vi "_FP Cntrl Manager.vi"(0 "Cluster":T1, 5 "Error IN":errorcluster, 8 "Action":T2) -> (19 "Error OUT":errorcluster)   [LabVIEW 2011]
uses:
  Controls/FP Ref Enum.ctl
  Controls/FP Ref Cluster.ctl
  Program Control/RS485 Settings Top Level.ctl
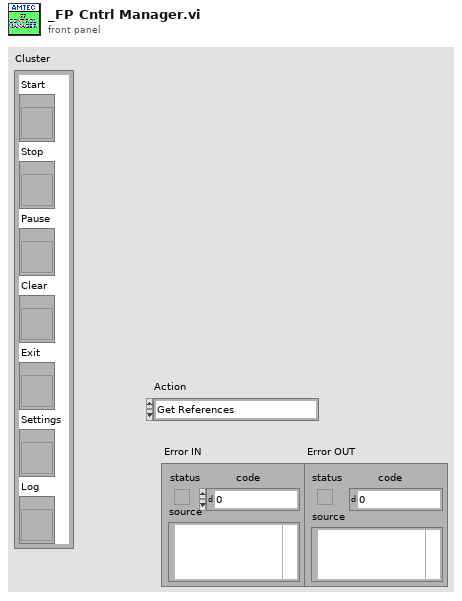
[diagram p1: front panel]
types:
  T1 = typedef "FP Ref Cluster.ctl" = cluster{"Start":refnum<vi>, "Stop":refnum<vi>, "Pause ":refnum<vi>, "Clear":refnum<vi>, "Exit":refnum<vi>, "Settings":refnum<vi>, "Log":refnum<vi>}
  T2 = typedef "FP Ref Enum.ctl" = enum16{"Get References", "Status", "Init", "Start Recording", "Stop Recording", "Pause Update", "Resume Update"}
  T3 = enum8{"Enabled", "Disabled", "Disabled and Grayed Out"}
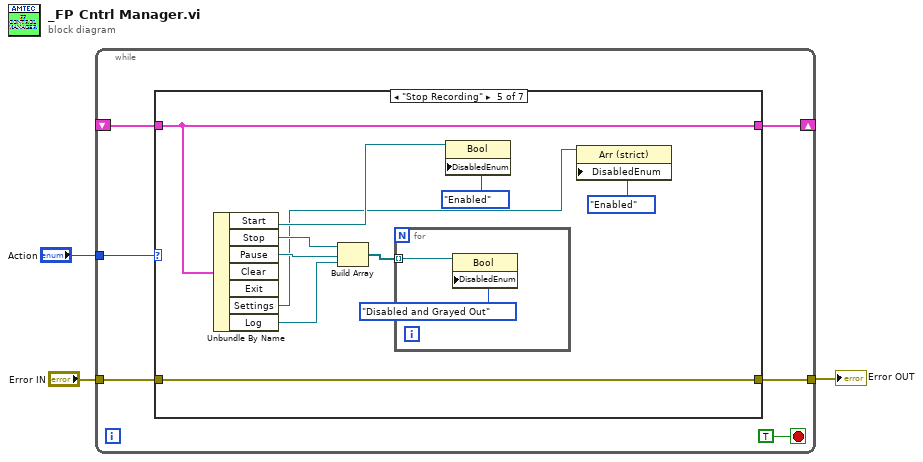
[diagram p0: block diagram]
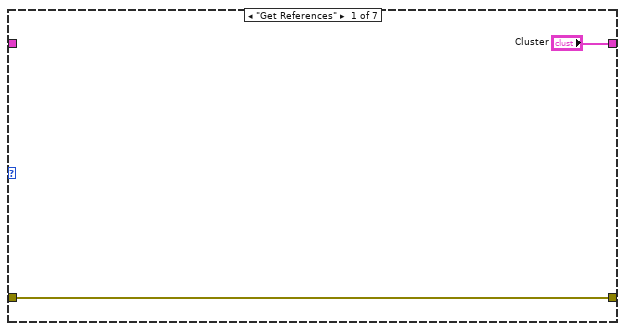
[diagram p2: hidden frame]
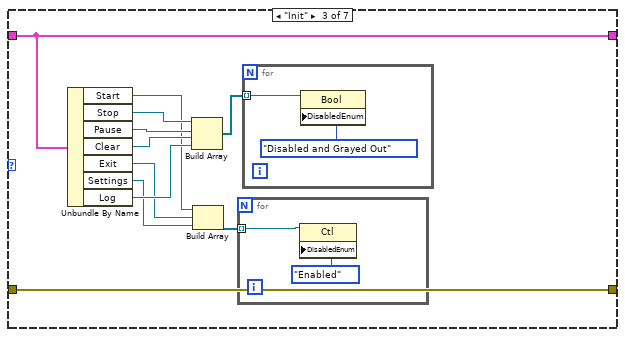
[diagram p4: hidden frame]
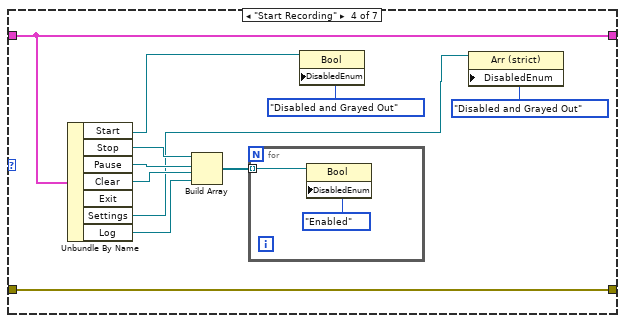
[diagram p5: hidden frame]
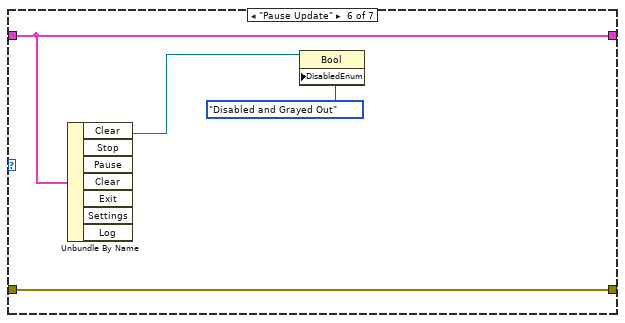
[diagram p6: hidden frame]
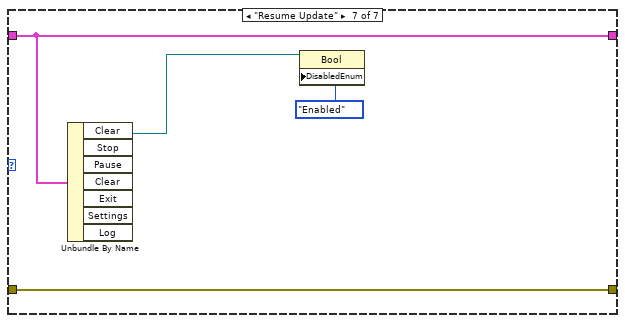
[diagram p7: hidden frame]
diagram:
  n1 = while {
    tunnel: "Action" -> [w8]
    tunnel: "Error IN" -> [w7]
    tunnel: [w6] -> w2
    shift-right: [w5] -> _
    shift-left: _ -> [w4]
    stop <- TRUE stop-if-true
    n2 = case shown="\"Stop Recording\"" w8 {
      tunnel: w7 -> [w11 w13 w24 w39 w51 w57 w61]
      tunnel: [w11 w13 w24 w39 w51 w57 w61] -> w6
      tunnel: ["Cluster" w12 w23 w38 w50 w56 w60] -> w5
      tunnel: w4 -> [_ w12 w23 w38 w50 w56 w60]
      frame "Get References" {
      }
      frame "Status", Default {
      }
      frame "Init" {
        n3 = Unbundle By Name(w23) -> ("Start"=w16:refnum<vi>, "Stop"=w22:refnum<vi>, "Pause"=w20:refnum<vi>, "Clear"=w19:refnum<vi>, "Exit"=w15:refnum<vi>, "Settings"=w14:refnum<vi>, "Log"=w21:refnum<vi>)
        n4 = Build Array(w22, w20, w19, w21) -> (w18:refnum<vi>[])
        n5 = Build Array(w16, w15, w14) -> (w17:refnum<vi>[])
        n6 = for {
          tunnel: w17 -> [w26] mode=indexing
          n7 = property class="Ctl"(reference=w26, "DisabledEnum"=T3."Enabled" ("Disabled")) -> ()  [unwired: 1 in, 2 out]
        }
        n8 = for {
          tunnel: w18 -> [w28] mode=indexing
          n9 = property class="Bool"(reference=w28, "DisabledEnum"=T3."Disabled and Grayed Out" ("Disabled")) -> ()  [unwired: 1 in, 2 out]
        }
      }
      frame "Start Recording" {
        n10 = Unbundle By Name(w38) -> ("Start"=w31:refnum<vi>, "Stop"=w37:refnum<vi>, "Pause"=w35:refnum<vi>, "Clear"=w34:refnum<vi>, "Settings"=w30:refnum<vi>, "Log"=w36:refnum<vi>)  [unwired: 1 out]
        n11 = Build Array(w37, w35, w34, w36) -> (w33:refnum<vi>[])
        n12 = for {
          tunnel: w33 -> [w41] mode=indexing
          n13 = property class="Bool"(reference=w41, "DisabledEnum"=T3."Enabled" ("Disabled")) -> ()  [unwired: 1 in, 2 out]
        }
        n14 = property class="Bool"(reference=w31, "DisabledEnum"=T3."Disabled and Grayed Out" ("Disabled")) -> ()  [unwired: 1 in, 2 out]
        n15 = property class="Arr (strict)"(reference=w30, "DisabledEnum"=T3."Disabled and Grayed Out" ("Disabled")) -> ()  [unwired: 1 in, 2 out]
      }
      frame "Stop Recording" {
        n16 = Unbundle By Name(w50) -> ("Start"=w44:refnum<vi>, "Stop"=w49:refnum<vi>, "Pause"=w47:refnum<vi>, "Settings"=w42:refnum<vi>, "Log"=w48:refnum<vi>)  [unwired: 2 out]
        n17 = Build Array(w49, w47, w48) -> (w46:refnum<vi>[])
        n18 = for {
          tunnel: w46 -> [w53] mode=indexing
          n19 = property class="Bool"(reference=w53, "DisabledEnum"=T3."Disabled and Grayed Out" ("Disabled")) -> ()  [unwired: 1 in, 2 out]
        }
        n20 = property class="Bool"(reference=w44, "DisabledEnum"=T3."Enabled" ("Disabled")) -> ()  [unwired: 1 in, 2 out]
        n21 = property class="Arr (strict)"(reference=w42, "DisabledEnum"=T3."Enabled" ("Disabled")) -> ()  [unwired: 1 in, 2 out]
      }
      frame "Pause Update" {
        n22 = Unbundle By Name(w56) -> ("Clear"=w54:refnum<vi>)  [unwired: 6 out]
        n23 = property class="Bool"(reference=w54, "DisabledEnum"=T3."Disabled and Grayed Out" ("Disabled")) -> ()  [unwired: 1 in, 2 out]
      }
      frame "Resume Update" {
        n24 = Unbundle By Name(w60) -> ("Clear"=w58:refnum<vi>)  [unwired: 6 out]
        n25 = property class="Bool"(reference=w58, "DisabledEnum"=T3."Enabled" ("Disabled")) -> ()  [unwired: 1 in, 2 out]
      }
    }
  }
  "Error OUT" <- w2
